vi "CC Script Parse Telescope Move RA DEC.vi"(8 "error in (no error)":errorcluster, 9 "To Script?":bool, 10 "RA and DEC":T1, 11 "Telescope Move Parameters":string="RA=14:29:33.123,DEC=090:15:22.110") -> (0 "error out":errorcluster, 2 "Script Out":string="ObjectName \"RA\":\"123.456\",\"DEC\":\"4546.54\"", 3 "RA and DEC":T1)   [LabVIEW 2024]
uses:
  typedefs/CC cluster RA and DEC.ctl
  <vilib>/regexp/Match Regular Expression.xnode
  Telescope/Telescope.lvclass
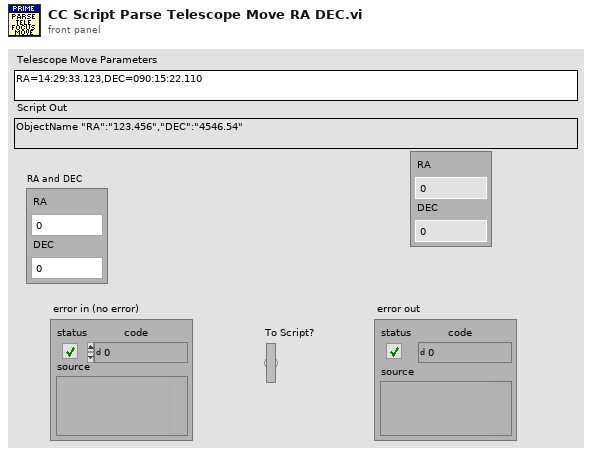
[diagram p1: front panel]
types:
  T1 = typedef "CC cluster RA and DEC.ctl" = cluster{"RA":dbl, "DEC":dbl}
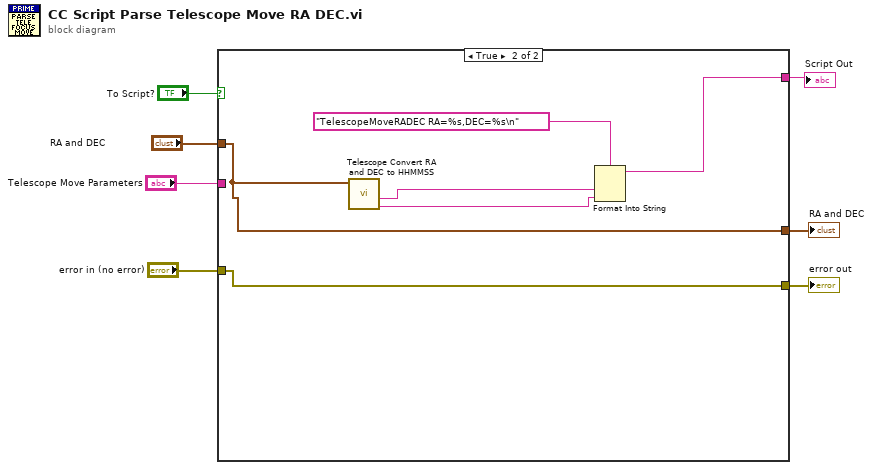
[diagram p0: block diagram]
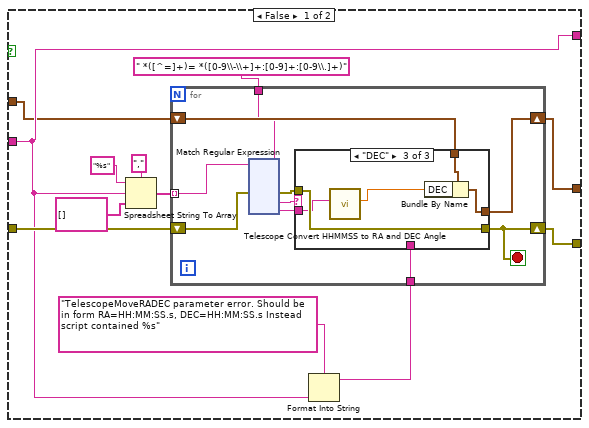
[diagram p2: hidden frame]
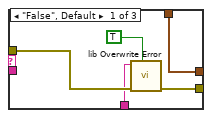
[diagram p3: hidden frame]
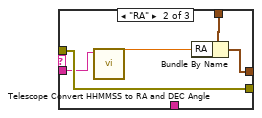
[diagram p4: hidden frame]
diagram:
  n1 = case shown="True" "To Script?" {
    tunnel: [w8 w167] -> w7
    tunnel: "error in (no error)" -> [w19 w168]
    tunnel: [w11 w168] -> w5
    tunnel: "Telescope Move Parameters" -> [w14 _]
    tunnel: "RA and DEC" -> [w9 w167]
    tunnel: [w14 w169] -> w2
    frame False {
      n2 = Spreadsheet String To Array(delimiter (Tab)=",", format string="%s", spreadsheet string=w14, array type (2D Dbl)=string[] []) -> (array=w13:string[])
      n3 = Format Into String(format string="TelescopeMoveRADEC parameter error. Should be in form RA=HH:MM:SS.s, DEC=HH:MM:SS.s Instead script contained %s", w14) -> (resulting string=w12:string)  [unwired: 2 in, 1 out]
      n4 = for {
        shift-right: [w28] -> w8
        shift-left: w9 -> [w29]
        tunnel: w13 -> [w27] mode=indexing
        tunnel: w12 -> [w22]
        shift-right: [w21] -> w11
        shift-left: w19 -> [w24]
        tunnel: " *([^=]+)= *([0-9\\-\\+]+:[0-9]+:[0-9\\.]+)" ("format string") -> [w20]
        stop <- w21 stop-if-true
        n5 = xnode "Match Regular Expression"("input string"=w27, "regular expression"=w20, "error in"=w24) -> ("error out"=w23:errorcluster, "submatch 1"=w26:string, "submatch 2"=w25:string)  [unwired: 3 in, 4 out]
        n6 = case shown="\"DEC\"" w26 {
          tunnel: w29 -> [w31 w37 w43]
          tunnel: [w31 w35 w42] -> w28
          tunnel: w25 -> [_ w38 w40]
          tunnel: w23 -> [w34 w39 w44]
          tunnel: w22 -> [w33 _ _]
          tunnel: [w32 w39 w44] -> w21
          frame "False", Default {
            n7 = call "lib Overwrite Error.vi"("Force Error?"=TRUE, "error in (no error)"=w34, "Error Message"=w33) -> ("error out"=w32:errorcluster)  [unwired: 8 in]
          }
          frame "RA" {
            n8 = call "Telescope Convert HHMMSS to RA and DEC Angle.vi"("RA String"=w38) -> ("RA"=w36:dbl)  [unwired: 8 in, 2 out]
            n9 = Bundle By Name(cluster=w37, "RA"=w36) -> (w35:T1)
          }
          frame "DEC" {
            n10 = call "Telescope Convert HHMMSS to RA and DEC Angle.vi"("Dec String"=w40) -> ("DEC"=w41:dbl)  [unwired: 8 in, 2 out]
            n11 = Bundle By Name(cluster=w43, "DEC"=w41) -> (w42:T1)
          }
        }
      }
    }
    frame True {
      n12 = call "Telescope Convert RA and DEC to HHMMSS.vi"("RA and DEC"=w167) -> ("Dec String"=w165:string, "RA String"=w166:string)  [unwired: 7 in, 2 out]
      n13 = Format Into String(format string="TelescopeMoveRADEC RA=%s,DEC=%s\n", w166, w165) -> (resulting string=w169:string)  [unwired: 2 in, 1 out]
    }
  }
  "error out" <- w5
  "RA and DEC" <- w7
  "Script Out" <- w2
